vi "Write Virtual Folder.vi"(10 "Virtual Folder":string, 11 "Test Runner.Project in":refnum<class "Test Runner.Project.lvclass">) -> (3 "Test Runner.Project out":refnum<class "Test Runner.Project.lvclass">)   [LabVIEW 2013, in "Caraya.lvlib" / "Test Runner.Project.lvclass"]
uses:
  Test Runner.Project.lvclass
  Test Runner.Project.lvclass/Test Runner.Project.ctl
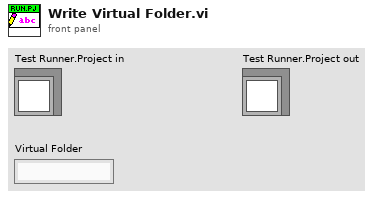
[diagram p1: front panel]
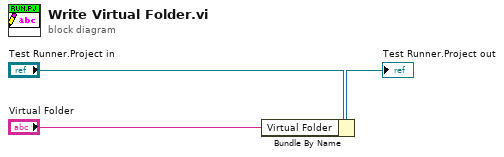
[diagram p0: block diagram]
diagram:
  n1 = Bundle By Name(cluster="Test Runner.Project in", "Virtual Folder"="Virtual Folder") -> (→"Test Runner.Project out":refnum<class "Test Runner.Project.lvclass">)
